vi "Table Buffer - Destroy.vi"(8 "error in (no error)":errorcluster) -> (0 "error out":errorcluster)   [LabVIEW 2025, in "I2C Bus Monitor UI.lvlib"]
uses:
  I2C Bus Monitor UI.lvlib
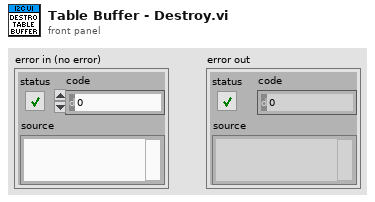
[diagram p1: front panel]
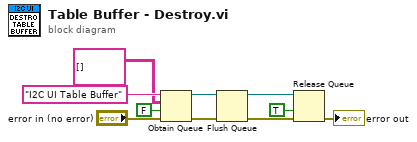
[diagram p0: block diagram]
diagram:
  n1 = Obtain Queue(name (unnamed)="I2C UI Table Buffer", element data type=string[][] [] ("I2C Messages"), create if not found? (T)=FALSE, error in (no error)="error in (no error)") -> (queue out=w2:refnum<queue>, error out=w8:errorcluster)  [unwired: 1 in, 1 out]
  n2 = Flush Queue(queue=w2, error in (no error)=w8) -> (queue out=w1:refnum<queue>, error out=w3:errorcluster)  [unwired: 1 out]
  n3 = Release Queue(queue=w1, force destroy? (F)=TRUE, error in (no error)=w3) -> (error out=→"error out":errorcluster)  [unwired: 2 out]
